vi "Fit VI window to Caller Center.vi"(4 "Error In":errorcluster, 6 "Background VI Ref (Callee's Caller)":refnum<vi>, 7 "VI Ref":refnum<vi>) -> (0 "Error Out":errorcluster, 3 "dup VI Ref":refnum<vi>)   [LabVIEW 2017, in "csm-ui-support.lvlib"]
doc: "This VI is designed to center a callee VI's window in a caller VI's window.\n\nAuthored by Brandon Steele\nsupport@mooregoodideas.com\nwww.mooregoodideas.com\n\nCopyright (c) 2010, Moore Good Ideas, Inc.\n\nAll rights reserved.\n\nRedistribution and use in source and binary forms, with or without modification, are permitted provided that the following conditions are met:\n\n * Redistributions of source code must retain the above copyright notice, this list of conditions and the following disclaimer.\n * Redistributions in binary form must reproduce the above copyright notice, this list of conditions and the following disclaimer in the documentation and/or other materials provided with the distribution.\n * Neither the name of Moore Good Ideas, Inc. nor the names of its contributors may be used to endorse or promote products derived from this software without specific prior written permission.\n\nTHIS SOFTWARE IS PROVIDED BY THE COPYRIGHT HOLDERS AND CONTRIBUTORS \"AS IS\" AND ANY EXPRESS OR IMPLIED WARRANTIES, INCLUDING, BUT NOT LIMITED TO, THE IMPLIED WARRANTIES OF MERCHANTABILITY AND FITNESS FOR A PARTICULAR PURPOSE ARE DISCLAIMED. IN NO EVENT SHALL THE COPYRIGHT OWNER OR CONTRIBUTORS BE LIABLE FOR ANY DIRECT, INDIRECT, INCIDENTAL, SPECIAL, EXEMPLARY, OR CONSEQUENTIAL DAMAGES (INCLUDING, BUT NOT LIMITED TO, PROCUREMENT OF SUBSTITUTE GOODS OR SERVICES; LOSS OF USE, DATA, OR PROFITS; OR BUSINESS INTERRUPTION) HOWEVER CAUSED AND ON ANY THEORY OF LIABILITY, WHETHER IN CONTRACT, STRICT LIABILITY, OR TORT (INCLUDING NEGLIGENCE OR OTHERWISE) ARISING IN ANY WAY OUT OF THE USE OF THIS SOFTWARE, EVEN IF ADVISED OF THE POSSIBILITY OF SUCH DAMAGE."
uses:
  csm-ui-support.lvlib
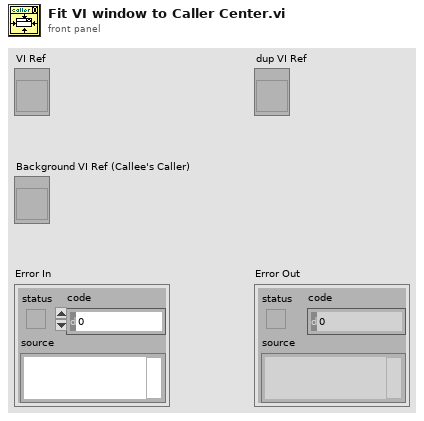
[diagram p1: front panel]
types:
  T1 = typedef "LVRectTypeDef.ctl" = cluster{"Left":i16, "Top":i16, "Right":i16, "Bottom":i16}
  T2 = cluster{"left":i16, "top":i16, "right":i16, "bottom":i16}
  T3 = typedef "LVAllMonitorsDisplayTypeDef.ctl" = cluster{"Bounds":cluster{"Left":i16, "Top":i16, "Right":i16, "Bottom":i16}, "Depth":i16}[]
  T4 = cluster{"Left":i16, "Top":i16, "Right":i16, "Bottom":i16}
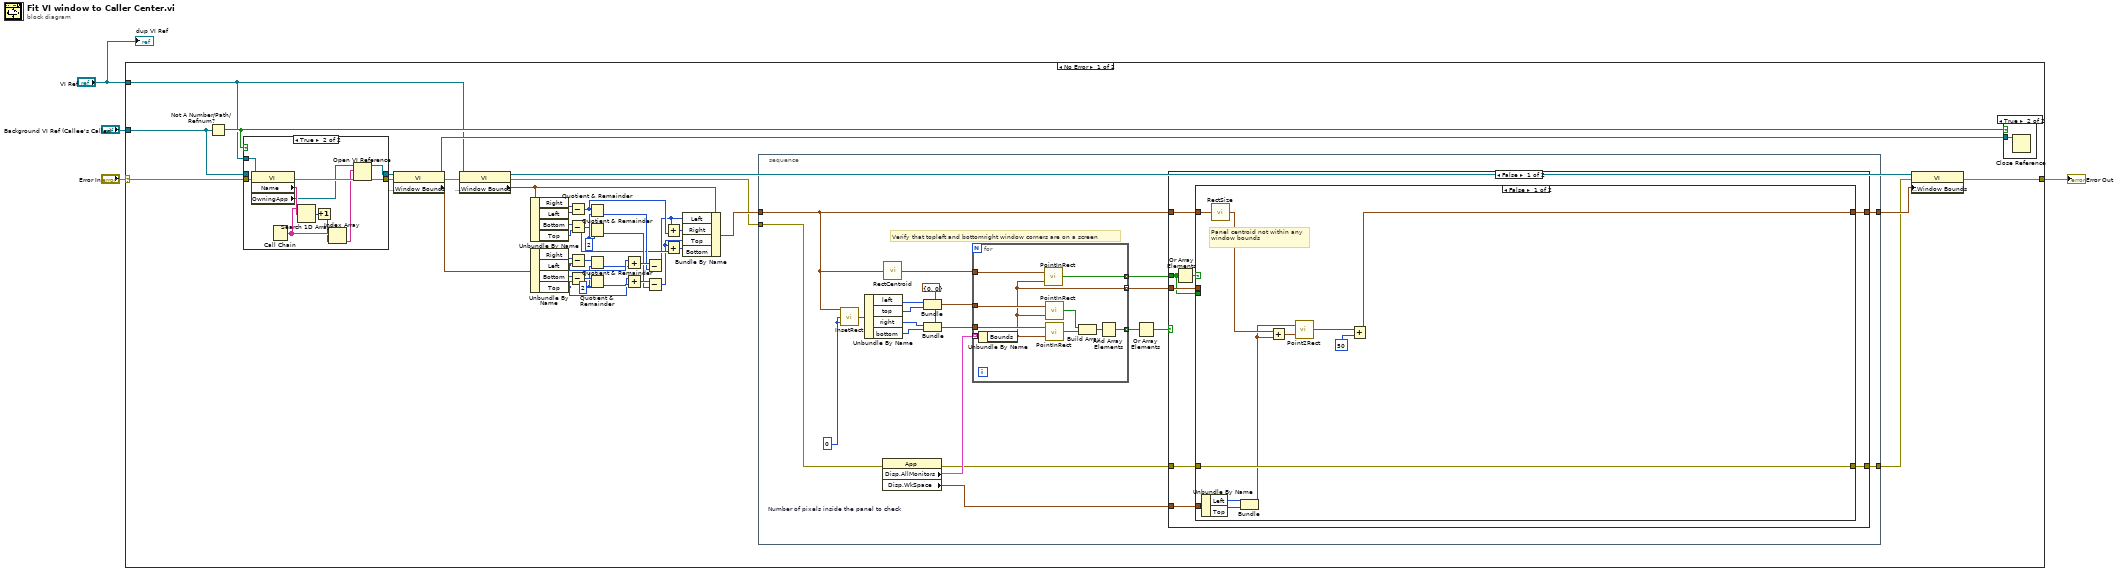
[diagram p0: block diagram]
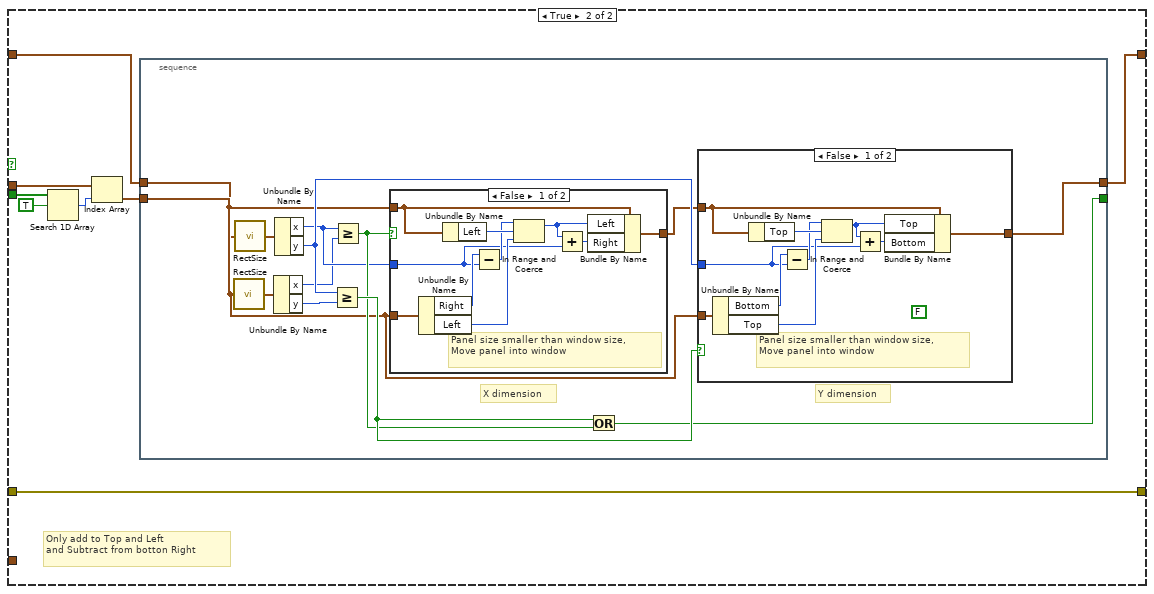
[diagram p2: hidden frame]
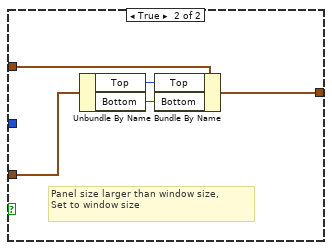
[diagram p3: hidden frame]
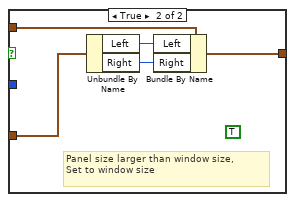
[diagram p4: hidden frame]
diagram:
  n1 = case shown="No Error" "Error In" {
    selector: "Error In" -> [w20 w162]
    tunnel: [w44 w162] -> w4
    tunnel: "Background VI Ref (Callee's Caller)" -> [w17 _]
    tunnel: "VI Ref" -> [w5 _]
    frame No Error {
      w37 = i16 2 ("y")
      w21 = i16 2 ("y")
      n2 = Not A Number/Path/Refnum?(number/path/refnum=w17) -> (NaN/Path/Refnum?=w18:bool)
      n3 = case shown="True" w18 {
        tunnel: w17 -> [w150 _]
        tunnel: [w150 w156] -> w16
        tunnel: w5 -> [_ w161]
        tunnel: w20 -> [w149 w160]
        tunnel: [w149 w157] -> w19
        frame False {
        }
        frame True {
          n4 = property class="VI"(reference=w161, error in=w160) -> (error out=w158:errorcluster, "Name"=w159:string, "OwningApp"=w153:refnum<vi>)  [unwired: 1 out]
          n5 = Call Chain() -> (call chain=w155:string[])
          n6 = Search 1D Array(1D array=w155, element=w159) -> (index of element=w152:i32)  [unwired: 1 in]
          n7 = Increment(x=w152) -> (x+1=w151:i32)
          n8 = Index Array(array=w155, index=w151) -> (element=w154:string)
          n9 = Open VI Reference(application reference (local)=w153, vi path=w154, error in (no error)=w158) -> (vi reference=w156:refnum<vi>, error out=w157:errorcluster)  [unwired: 3 in]
        }
      }
      n10 = property class="VI"(reference=w16, error in=w19) -> (reference out=w15:refnum<vi>, error out=w38:errorcluster, "Front Panel Window:Window Bounds"=w43:T1)
      n11 = property class="VI"(reference=w5, error in=w38) -> (reference out=w24:refnum<vi>, error out=w7:errorcluster, "Front Panel Window:Window Bounds"=w10:T1)
      n12 = Unbundle By Name(w10) -> ("Right"=w33:i16, "Left"=w34:i16, "Bottom"=w35:i16, "Top"=w36:i16)
      n13 = Unbundle By Name(w43) -> ("Right"=w42:i16, "Left"=w32:i16, "Bottom"=w41:i16, "Top"=w29:i16)
      n14 = Subtract(x=w33, y=w34) -> (x-y=w23:i16)
      n15 = Subtract(x=w35, y=w36) -> (x-y=w22:i16)
      n16 = Subtract(x=w42, y=w32) -> (x-y=w40:i16)
      n17 = Subtract(x=w41, y=w29) -> (x-y=w39:i16)
      n18 = Quotient & Remainder(x=w23, y=w37) -> (floor(x/y)=w27:i16)  [unwired: 1 out]
      n19 = Quotient & Remainder(x=w22, y=w37) -> (floor(x/y)=w25:i16)  [unwired: 1 out]
      n20 = Quotient & Remainder(x=w40, y=w21) -> (floor(x/y)=w31:i16)  [unwired: 1 out]
      n21 = Quotient & Remainder(x=w39, y=w21) -> (floor(x/y)=w30:i16)  [unwired: 1 out]
      n22 = Add(x=w32, y=w31) -> (x+y=w28:i16)
      n23 = Add(x=w29, y=w30) -> (x+y=w26:i16)
      n24 = Subtract(x=w28, y=w27) -> (x-y=w13:i16)
      n25 = Subtract(x=w26, y=w25) -> (x-y=w12:i16)
      n26 = Add(x=w13, y=w23) -> (x+y=w11:i16)
      n27 = Add(x=w12, y=w22) -> (x+y=w14:i16)
      n28 = Bundle By Name(cluster=w10, "Left"=w13, "Right"=w11, "Top"=w12, "Bottom"=w14) -> (w9:T1)
      n29 = stacked-sequence {
        tunnel: [w55] -> w6
        tunnel: [w46] -> w8
        tunnel: w7 -> [w48]
        tunnel: w9 -> [w62]
        frame #0 {
          w57 = i16 0  # Number of pixels inside the panel to check
          w61 = cluster{"x":i16, "y":i16} {"x"=0, "y"=0} ("point")
          # "Verify that topleft and bottomright window corners are on a screen"
          n30 = call <vilib>:"InsetRect.vi"("dv"=w57, "dh"=w57, "rect"=w62) -> ("inset rect"=w51:T2)
          n31 = Unbundle By Name(w51) -> ("left"=w49:i16, "top"=w50:i16, "right"=w58:i16, "bottom"=w59:i16)
          n32 = property class="App"(error in=w48) -> (error out=w45:errorcluster, "Disp.AllMonitors"=w47:T3, "Disp.WkSpace"=w56:T1)  [unwired: 1 in, 1 out]
          n33 = call <vilib>:"RectCentroid.vi"("rect"=w62) -> ("point"=w63:cluster{"x":i16, "y":i16})
          n34 = Bundle(cluster=w61, "x"=w49, "y"=w50) -> (w52:cluster{"x":i16, "y":i16})
          n35 = Bundle(cluster=w61, "x"=w58, "y"=w59) -> (w60:cluster{"x":i16, "y":i16})
          n36 = for {
            tunnel: w47 -> [w147] mode=indexing
            tunnel: w52 -> [w146]
            tunnel: [w142] -> w53 mode=indexing
            tunnel: w60 -> [w141]
            tunnel: w63 -> [w140]
            tunnel: [w139] -> w64 mode=indexing
            tunnel: [w138] -> w65 mode=indexing
            n37 = Unbundle By Name(w147) -> ("Bounds"=w138:T4)
            n38 = call <vilib>:"PointInRect.vi"("rect"=w138, "point"=w140) -> ("pt in rect"=w139:bool)
            n39 = call <vilib>:"PointInRect.vi"("rect"=w138, "point"=w146) -> ("pt in rect"=w145:bool)
            n40 = call <vilib>:"PointInRect.vi"("rect"=w138, "point"=w141) -> ("pt in rect"=w144:bool)
            n41 = Build Array(w145, w144) -> (w143:bool[])
            n42 = And Array Elements(Boolean array=w143) -> (logical AND=w142:bool)
          }
          n43 = Or Array Elements(Boolean array=w53) -> (logical OR=w54:bool)
          n44 = case shown="False" w54 {
            tunnel: w45 -> [w68 w137]
            tunnel: [w67 w137] -> w55
            tunnel: w62 -> [w72 w136]
            tunnel: [w71 w136] -> w46
            tunnel: w56 -> [w73 _]
            tunnel: w64 -> [w66 _]
            tunnel: w65 -> [w69 _]
            frame False {
              n45 = Or Array Elements(Boolean array=w66) -> (logical OR=w70:bool)
              n46 = case shown="False" w70 {
                tunnel: w73 -> [w84 _]
                tunnel: w72 -> [w80 w87]
                tunnel: [w78 w85] -> w71
                tunnel: w69 -> [_ w89]
                tunnel: w68 -> [w77 w92]
                tunnel: [w77 w92] -> w67
                tunnel: w66 -> [_ w91]
                frame False {
                  # "Panel centroid not within any\nwindow bounds"
                  n47 = Unbundle By Name(w84) -> ("Left"=w83:i16, "Top"=w82:i16)
                  n48 = call <vilib>:"RectSize.vi"("rect"=w80) -> ("point"=w76:cluster{"x":i16, "y":i16})
                  n49 = Bundle("Left"=w83, "Top"=w82) -> (w74:cluster{"Left":i16, "Top":i16})  [unwired: 1 in]
                  n50 = Add(x=w76, y=w74) -> (x+y=w75:cluster{i16, i16})
                  n51 = call <vilib>:"Point2Rect.vi"("point b"=w75, "point a"=w74) -> ("rect"=w79:T2)
                  n52 = Add(x=w79, y=i16 50) -> (x+y=w78:T2)
                }
                frame True {
                  # "Only add to Top and Left\nand Subtract from botton Right"
                  n53 = Search 1D Array(1D array=w91, element=TRUE) -> (index of element=w88:i32)  [unwired: 1 in]
                  n54 = Index Array(array=w89, index=w88) -> (element=w86:T4)
                  n55 = stacked-sequence {
                    tunnel: [w93] -> _
                    tunnel: [w103] -> w85
                    tunnel: w86 -> [w102]
                    tunnel: w87 -> [w94]
                    frame #0 {
                      # "X dimension"
                      # "Y dimension"
                      n56 = call <vilib>:"RectSize.vi"("rect"=w102) -> ("point"=w96:cluster{"x":i16, "y":i16})
                      n57 = call <vilib>:"RectSize.vi"("rect"=w94) -> ("point"=w95:cluster{"x":i16, "y":i16})
                      n58 = Unbundle By Name(w96) -> ("x"=w97:i16, "y"=w100:i16)
                      n59 = Unbundle By Name(w95) -> ("x"=w98:i16, "y"=w101:i16)
                      n60 = Greater Or Equal?(x=w101, y=w100) -> (x >= y?=w105:bool)
                      n61 = Greater Or Equal?(x=w98, y=w97) -> (x >= y?=w104:bool)
                      n62 = case shown="False" w104 {
                        tunnel: w102 -> [w130 w131]
                        tunnel: w94 -> [w122 w132]
                        tunnel: w98 -> [w123 _]
                        tunnel: [w121 w133] -> w99
                        frame False {
                          # "Panel size smaller than window size,\nMove panel into window"
                          n63 = Unbundle By Name(w130) -> ("Right"=w126:i16, "Left"=w128:i16)
                          n64 = Unbundle By Name(w122) -> ("Left"=w129:i16)
                          n65 = Subtract(x=w126, y=w123) -> (x-y=w127:i16)
                          n66 = In Range and Coerce(upper limit=w127, x=w129, lower limit=w128) -> (coerced(x)=w125:i16)  [unwired: 1 out]
                          n67 = Add(x=w125, y=w123) -> (x+y=w124:i16)
                          n68 = Bundle By Name(cluster=w122, "Left"=w125, "Right"=w124) -> (w121:T1)
                        }
                        frame True {
                          (unwired) TRUE
                          # "Panel size larger than window size,\nSet to window size"
                          n69 = Unbundle By Name(w131) -> ("Left"=w135:i16, "Right"=w134:i16)
                          n70 = Bundle By Name(cluster=w132, "Left"=w135, "Right"=w134) -> (w133:T1)
                        }
                      }
                      n71 = Or(x=w105, y=w104) -> (x .or. y?=w93:bool)
                      n72 = case shown="False" w105 {
                        tunnel: w102 -> [w115 w120]
                        tunnel: w99 -> [w107 w116]
                        tunnel: w101 -> [w108 _]
                        tunnel: [w106 w117] -> w103
                        frame False {
                          (unwired) FALSE
                          # "Panel size smaller than window size,\nMove panel into window"
                          n73 = Unbundle By Name(w115) -> ("Bottom"=w111:i16, "Top"=w113:i16)
                          n74 = Unbundle By Name(w107) -> ("Top"=w114:i16)
                          n75 = Subtract(x=w111, y=w108) -> (x-y=w112:i16)
                          n76 = In Range and Coerce(upper limit=w112, x=w114, lower limit=w113) -> (coerced(x)=w110:i16)  [unwired: 1 out]
                          n77 = Add(x=w110, y=w108) -> (x+y=w109:i16)
                          n78 = Bundle By Name(cluster=w107, "Top"=w110, "Bottom"=w109) -> (w106:T1)
                        }
                        frame True {
                          # "Panel size larger than window size,\nSet to window size"
                          n79 = Unbundle By Name(w120) -> ("Top"=w119:i16, "Bottom"=w118:i16)
                          n80 = Bundle By Name(cluster=w116, "Top"=w119, "Bottom"=w118) -> (w117:T1)
                        }
                      }
                    }
                  }
                }
              }
            }
            frame True {
            }
          }
        }
      }
      n81 = property class="VI"(reference=w24, error in=w6, "Front Panel Window:Window Bounds"=w8) -> (error out=w44:errorcluster)  [unwired: 1 out]
      n82 = case shown="True" w18 {
        tunnel: w15 -> [_ w148]
        frame False {
        }
        frame True {
          n83 = Close Reference(reference=w148) -> ()  [unwired: 1 in, 1 out]
        }
      }
    }
    frame Error {
    }
  }
  "Error Out" <- w4
  "dup VI Ref" <- "VI Ref"
